vi "FPGA_HoppingScan_CircularBuffered.vi"() -> ()   [LabVIEW 2024]
uses:
  <vilib>/Platform/TimedLoop/XDataNode/timing_clust.ctl
  <vilib>/Platform/TimedLoop/XDataNode/nitl_modes.ctl
  <vilib>/Platform/TimedLoop/XDataNode/wakeup.ctl
  <vilib>/rvi/FXPMathLib/FxpDiv/subVIs/nifxpmath_Div_SimConfig.ctl
  <vilib>/rvi/Emulation/niFpgaSctlEmulationGetInTimedLoop.vi
  <vilib>/rvi/Emulation/niFpgaProcessEmulError.vi
  <vilib>/rvi/Memory/Memory_Emulation/nirvimemoryFastEmulation.vi
  <vilib>/rvi/Memory/Memory_Emulation/nirvimemoryEmulation.vi
  <vilib>/rvi/Emulation/niFpgaEmulationIsFPGAContextNoSignature.vi
  <vilib>/rvi/DataTransferAndStorage/Container/Common/niFpgaContainerGetUniqueNameForEmu.vi
  <vilib>/rvi/errors/nirviReportUnexpectedCaseInternalError (U32).vi
  <vilib>/rvi/eio/common/nirviEmuTemplateMethod_errors.vi
  <vilib>/rvi/Emulation/niFpgaEmulationReportErrorSimple.vi
  <vilib>/rvi/Emulation/niFpgaGetClockAttributes.vi
  <vilib>/rvi/Emulation/niFpgaCriticalErrorInLSC.vi
  <vilib>/rvi/Memory/Memory_Emulation/niFpgaMemoryEmulationCacheClearOnFirstRun.vi
  <vilib>/rvi/Memory/Memory_Emulation/nirvimemoryEmulationManagerCache_MakeExclusive.vi
  <vilib>/rvi/Memory/Memory_Emulation/niFpgaMemoryEmulationValidateCache.vi
  <vilib>/rvi/Memory/Memory_Emulation/nirvimemoryEmulationManagerCache_InsertValue.vi
  <vilib>/Utility/error.llb/Clear Errors.vi
  <vilib>/rvi/Memory/Memory_Emulation/nirvimemoryEmulationManagerCache_ReleaseExclusive.vi
  <vilib>/rvi/Memory/Memory_Emulation/nirvimemoryEmulationManagerCache_GetValue.vi
  <vilib>/rvi/Memory/Memory_Emulation/nirvimemoryEmulationManagerCache_SetValue.vi
  <vilib>/rvi/FIFO/Fifo_Resource/nirvififoEmulationSetSize.vi
  <vilib>/rvi/FIFO/Fifo_Resource/nirviFifoEmulationQueueMgr.vi
  <instcachedir>/0/nirviFifoEmulationQueueMgr_E5CAEC123FF24DC58D834DCA3CDAA9B5.lvgen/nirviFifoEmulationQueueMgr_E5CAEC123FF24DC58D834DCA3CDAA9B5_001.vi
  <vilib>/rvi/errors/niFpgaSetErrorForExecOnDevCompSimple.vi
  <vilib>/rvi/eio/common/nirviEmuReportErrorAndStop.vi
  <vilib>/rvi/FIFO/Fifo_Resource/nirvififoEmulationCreateLock.vi
  <vilib>/rvi/FIFO/Fifo_Resource/nirvififoEmulationObtainLock.vi
  <vilib>/rvi/FIFO/Fifo_Resource/nirvififoEmulationReleaseLock.vi
  <vilib>/rvi/occurrence/nirviWaitOnOccurrenceBase.vi
  <vilib>/rvi/errors/nirviReportUnexpectedCaseInternalError.vi
  <vilib>/eio/utilities/niEioResolveVilibRelativePath.vi
  <vilib>/rvi/interface/RandomDataEmulation/niFpgaRandomDataHandleErrors.vi
  <vilib>/rvi/FXPMathLib/FxpDiv/simVIs/DllFxpDivTemp_sub.vi
  <vilib>/rvi/FIFO/Fifo_Resource/nirvififoEmulationDetermineInputValidOut.vi
  <vilib>/rvi/DataTransferAndStorage/Container/XNode/niFpgaContainer.xnode
  <vilib>/eio/EIONode/EIONode.xnode
  <vilib>/platform/TimedLoop/XDataNode/XDataNode.xnode
  <vilib>/rvi/DataTransferAndStorage/Register/Emulation/niFpgaRegisterEmulation.vi
  <vilib>/rvi/FIFO/Fifo_Resource/nirvififoEmulationGetNumberOfElementsToRead.vi
  <vilib>/rvi/FIFO/Fifo_Resource/nirvififoEmulationRead.vi
  <vilib>/rvi/interface/RandomDataEmulation/nirviRandomDataFpgaReadWriteTemplate.vi
  <vilib>/rvi/FXPMathLib/FxpSub/XNode/nifxpmath_Sub.xnode
  <vilib>/rvi/FXPMathLib/FxpAdd/XNode/nifxpmath_Add.xnode
  <vilib>/rvi/FXPMathLib/FxpMul/XNode/nifxpmath_Multiplier.xnode
  <vilib>/rvi/FXPMathLib/FxpDiv/XNode/nifxpmath_Div.xnode
  <vilib>/rvi/FIFO/Fifo_Resource/nirvififoEmulationWrite.vi
  <vilib>/rvi/FXPMathLib/sim/FxpSim.dll
  <vilib>/Platform/TimedLoop/XDataNode/XDNodeRunTimeDep.lvlib
panel:
  in  "DelayPoints":i32
  in  "Halting Threshold":fxp<+/-,48,16>
  out "point_scanned":u32
  in  "TotalPoints":u32
  in  "RetRate us":i32
  in  "AppRate_NF us":i32
  in  "AppRate_FF us":i32
  in  "Recording Threshold":fxp<+/-,48,16>
  in  "stop":bool
  out "TargetDone?":bool
  out "ScanFinished?":bool
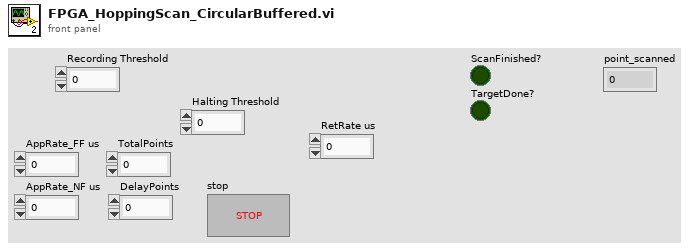
[diagram p1: front panel]
types:
  T1 = typedef "XDNodeRunTimeDep.lvlib/timing_clust.ctl" = cluster{"Expected End [f-1]":u64, "Actual End [f-1]":u64, "Finished Late? [f-1]":bool, "Expected End [i-1]":u64, "Actual End [i-1]":u64, "Finished Late? [i-1]":bool, "Expected Start [i]":u64, "Actual Start [i]":u64, "Expected Start [f]":u64, "Actual Start [f]":u64, "Source Name":string, "Structure Name":string, "Period":i64, "Deadline":i64, "Offset":i64, "Start":i64, "Priority":i32, "Timeout":i32, "Mode":T2, "Wakeup Reason":T3, "Error":errorcluster, "Source Type":string, "Secondary Source Type":string, "Global End Time":u64, "Global Start Time":u64, "Frame Duration":u64, "Iteration Duration":u64, "Assigned CPU":i32, "I/O Scan Engine Mode":u32}
  T2 = typedef "XDNodeRunTimeDep.lvlib/nitl_modes.ctl" = enum32{"No Change", "Process missed periods, maintain original phase", "Discard missed periods, maintain original phase", "Process missed periods, ignore original phase", "Discard missed periods, ignore original phase"}
  T3 = typedef "XDNodeRunTimeDep.lvlib/wakeup.ctl" = enum32{"Normal", "Aborted", "Asynchronous wakeup", "Timing source error", "Timed loop error", "Timeout"}
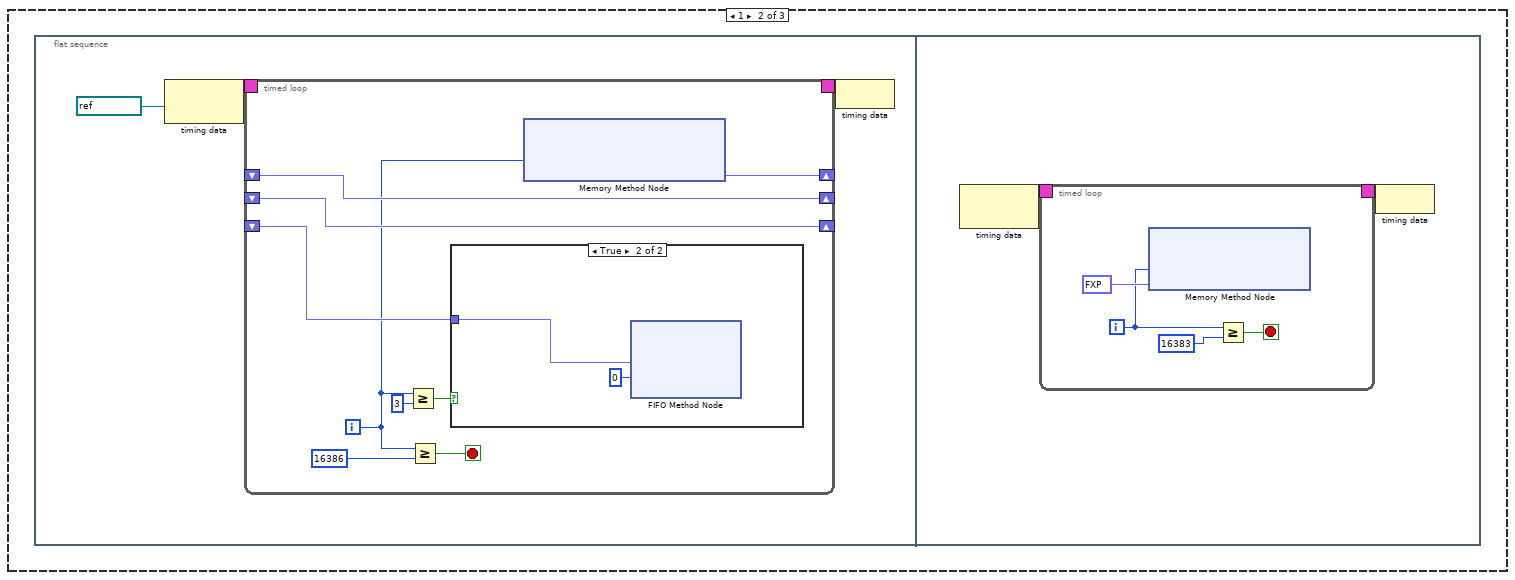
[diagram p4: hidden frame]
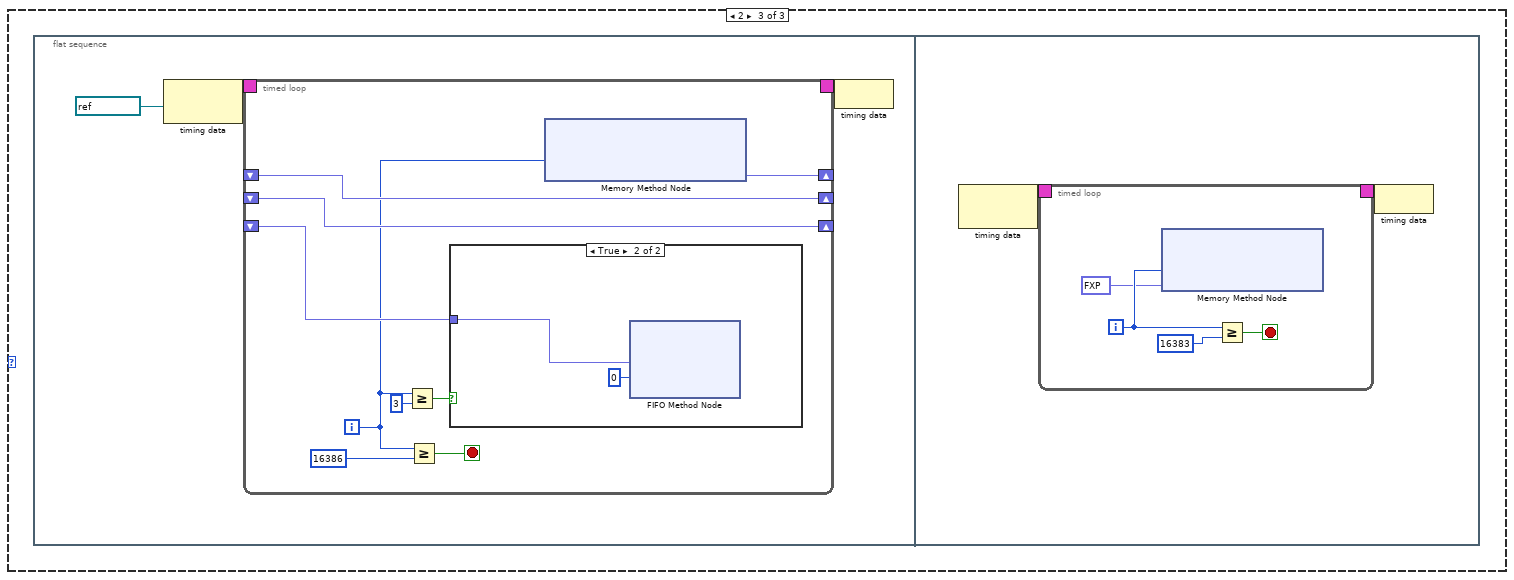
[diagram p6: hidden frame]
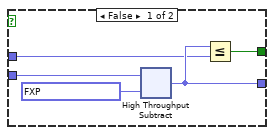
[diagram p13: hidden frame]
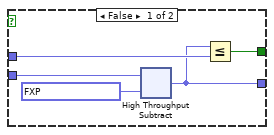
[diagram p14: hidden frame]
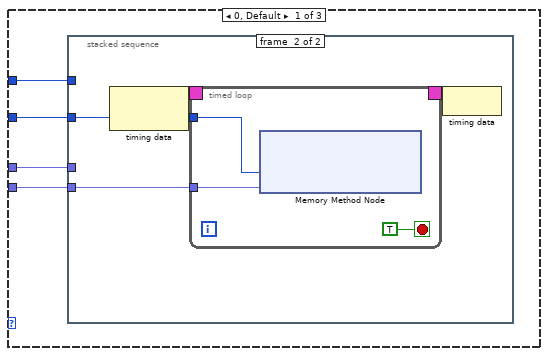
[diagram p16: hidden frame]
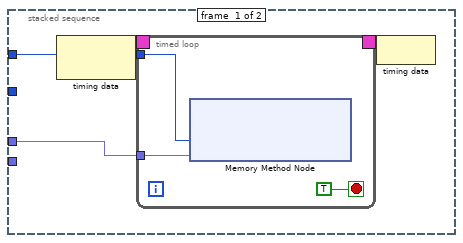
[diagram p17: hidden frame]
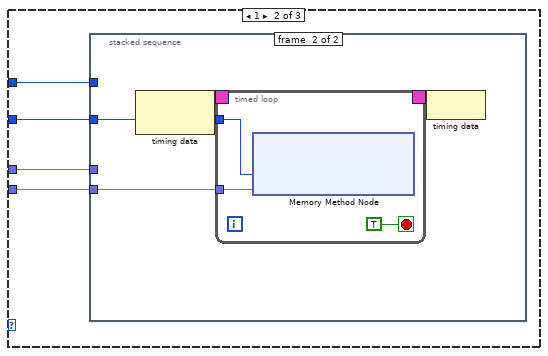
[diagram p18: hidden frame]
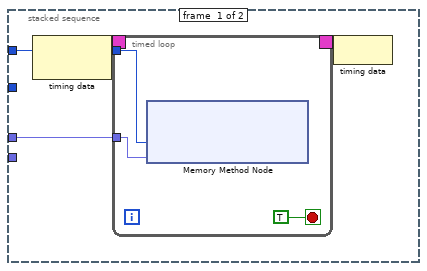
[diagram p19: hidden frame]
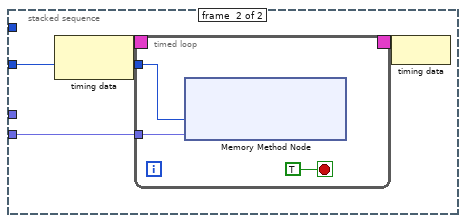
[diagram p20: hidden frame]
diagram:
  n1 = flat-sequence {
    tunnel: [w18] -> w1
    tunnel: w1 -> [w31]
    frame #0 {
      w7 = fxp<+/-,20,5> 0.0 ("Connector0/AO0")
      n2 = node-c288() -> (w3:T1)  [unwired: 1 in]
      n3 = timed-loop {
        timing: w3 -> [_]
        timing-out: [_] -> w2
        i -> [w9]
        stop <- w8 stop-if-true
        w11 = fxp<+/-,48,16> -100.0 ("Data")
        n4 = xnode ("Memory Method Node")("Address"=w9, "Data"=w11) -> ()  [unwired: 1 in, 1 out]
        n5 = xnode ("Memory Method Node")("Address"=w9, "Data"=w11) -> ()  [unwired: 1 in, 1 out]
        n6 = xnode ("Memory Method Node")("Address"=w9, "Data"=w11) -> ()  [unwired: 1 in, 1 out]
        n7 = Greater Or Equal?(x=w9, y=16383) -> (x >= y?=w8:bool)
      }
      n8 = for {
        N: 6 -> [_]
        i -> [w17]
        n9 = xnode ("Memory Method Node")("Address"=w17, "Data"=fxp<+/-,48,16> 0.0) -> ()  [unwired: 1 in, 1 out]
      }
      n10 = xnode "FPGA I/O Node"("Connector0/AO0"=w7, "Connector0/AO1"=w7, "Connector0/AO2"=w7) -> ()  [unwired: 3 in, 3 out]
      n11 = node-c288(w2) -> ()
      "ScanFinished?" <- FALSE
      "TargetDone?" <- FALSE
    }
    frame #1 {
      n12 = Generate Occurrence() -> (w18:refnum<k4>)
      n13 = call "Wait"("Count(mSec)"=u8 120) -> ()  [unwired: 1 out]
    }
    frame #2 {
      n14 = while {
        tunnel: w31 -> [w148]
        stop <- w150 stop-if-true
        n15 = xnode ("Register Read")() -> ("Data"=w151:bool)  [unwired: 1 in, 1 out]
        n16 = xnode ("FIFO Method Node")() -> ("Number of Elements to Read"=w154:u32)  [unwired: 1 in, 1 out]
        n17 = local read "ScanFinished?"() -> (w149:bool)
        n18 = Or(x=w151, y=w149) -> (x .or. y?=w150:bool)
        n19 = Greater Or Equal?(x=w154, y=u32 6) -> (x >= y?=w152:bool)
        n20 = case shown="True" w152 {
          tunnel: w148 -> [_ w155]
          frame False {
          }
          frame True {
            n21 = First Call?() -> (First Call?: T/F=w156:bool)
            n22 = case shown="True" w156 {
              tunnel: w155 -> [_ w157]
              frame False {
              }
              frame True {
                n23 = flat-sequence {
                  tunnel: [w160] -> w158
                  tunnel: w157 -> [w160]
                  tunnel: w158 -> [w161]
                  frame #0 {
                    n24 = call "Wait3"("Count(mSec)"=u8 4) -> ()  [unwired: 1 out]
                  }
                  frame #1 {
                    n25 = Set Occurrence(w161) -> ()
                  }
                }
              }
            }
          }
        }
      }
      n26 = while {
        tunnel: w31 -> [w133]
        stop <- w130 stop-if-true
        n27 = flat-sequence {
          tunnel: ["stop"] -> w135
          tunnel: w133 -> [w137]
          tunnel: [w137] -> w131
          tunnel: w135 -> [w140]
          tunnel: [w140] -> w134
          tunnel: [w139] -> w132
          tunnel: w131 -> [w139]
          tunnel: w134 -> [w144]
          tunnel: w132 -> [w143]
          tunnel: [w142] -> w130
          frame #0 {
            n28 = case shown="True" "stop" {
              tunnel: "stop" -> [_ w138]
              frame False {
              }
              frame True {
                n29 = xnode ("Register Write")("Data"=w138) -> ()  [unwired: 1 in, 1 out]
              }
            }
          }
          frame #1 {
            n30 = call "Wait2"("Count(uSec)"=u8 200) -> ()  [unwired: 1 out]
          }
          frame #2 {
            n31 = xnode ("Register Read")() -> ("Data"=w145:bool)  [unwired: 1 in, 1 out]
            n32 = local read "ScanFinished?"() -> (w146:bool)
            n33 = Compound Arithmetic op=OR(w146, w145, w144) -> (w142:bool)
            n34 = case shown="True" w142 {
              tunnel: w143 -> [_ w147]
              frame False {
              }
              frame True {
                n35 = Set Occurrence(w147) -> ()
              }
            }
          }
        }
      }
      n36 = flat-sequence {
        tunnel: w31 -> [w162]
        tunnel: [fxp<+/-,48,16> 0.0 ("Threshold")] -> w30
        tunnel: [w164] -> w28
        tunnel: [u8 0] -> w25
        tunnel: w30 -> [w167]
        tunnel: [w168] -> w29
        tunnel: w28 -> [w168]
        tunnel: [w167] -> w27
        tunnel: [w166] -> w26
        tunnel: w25 -> [w166]
        tunnel: w29 -> [w173]
        tunnel: w27 -> [w172]
        tunnel: w26 -> [w171]
        tunnel: [w170] -> w24
        tunnel: w24 -> [w1125]
        tunnel: [w1123] -> w23
        tunnel: [w1122] -> w21
        tunnel: w23 -> [w1137]
        tunnel: [w1137] -> w22
        tunnel: w21 -> [w1136]
        tunnel: [w1136] -> w20
        tunnel: w22 -> [w1141]
        tunnel: w20 -> [w1138]
        frame #0 {
          n37 = Wait on Occurrence(2:w162) -> ()  [unwired: 2 in, 1 out]
        }
        frame #1 {
          # "z piezo voltage"
          # "Swapchain indicator"
          n38 = xnode ("Register Read")() -> ("Data"=w164:bool)  [unwired: 1 in, 1 out]
        }
        frame #2 {
          n39 = call "Wait4"("Count(mSec)"=u8 4) -> ()  [unwired: 1 out]
        }
        frame #3 {
          n40 = case shown="False" w173 {
            tunnel: w172 -> [w176 w1121]
            tunnel: w171 -> [w175 _]
            tunnel: [w174 w1121] -> w170
            frame False {
              n41 = while {
                shift-right: [w184] -> w174
                shift-left: w176 -> [w218]
                shift-right: [w183] -> _
                shift-left: w175 -> [w197]
                stop <- w182 stop-if-true
                n42 = flat-sequence {
                  tunnel: w218 -> [w220]
                  tunnel: [w222] -> w217
                  tunnel: [w221] -> w213
                  tunnel: [w220] -> w202
                  tunnel: w197 -> [w219]
                  tunnel: [w219] -> w196
                  tunnel: w217 -> [w230]
                  tunnel: [w230] -> w216
                  tunnel: w213 -> [w229]
                  tunnel: [w229] -> w212
                  tunnel: w202 -> [w228]
                  tunnel: [w228] -> w201
                  tunnel: w196 -> [w227]
                  tunnel: [w227] -> w195
                  tunnel: w216 -> [w257]
                  tunnel: [w257] -> w215
                  tunnel: [w250] -> w214
                  tunnel: w212 -> [w256]
                  tunnel: [w256] -> w211
                  tunnel: [w251] -> w209
                  tunnel: [w254] -> w207
                  tunnel: [w253] -> w206
                  tunnel: [w252] -> w205
                  tunnel: w201 -> [w249]
                  tunnel: w195 -> [w255]
                  tunnel: [w255] -> w194
                  tunnel: [w246] -> w181
                  tunnel: [w248] -> w177
                  tunnel: w215 -> [w293]
                  tunnel: w214 -> [w294]
                  tunnel: w211 -> [w292]
                  tunnel: [w292] -> w210
                  tunnel: w209 -> [w291]
                  tunnel: [w291] -> w208
                  tunnel: w207 -> [w290]
                  tunnel: w206 -> [w288]
                  tunnel: w205 -> [w287]
                  tunnel: [w290] -> w204
                  tunnel: [w285] -> w200
                  tunnel: w194 -> [w289]
                  tunnel: [w289] -> w193
                  tunnel: [w288] -> w190
                  tunnel: [w287] -> w189
                  tunnel: w181 -> [w286]
                  tunnel: [w286] -> w180
                  tunnel: w177 -> [w285]
                  tunnel: w210 -> [w321]
                  tunnel: w208 -> [w322]
                  tunnel: w204 -> [w320]
                  tunnel: [w320] -> w203
                  tunnel: w200 -> [w319]
                  tunnel: [w319] -> w199
                  tunnel: w193 -> [w318]
                  tunnel: [w318] -> w191
                  tunnel: w190 -> [w317]
                  tunnel: w189 -> [w316]
                  tunnel: [w317] -> w188
                  tunnel: [w316] -> w187
                  tunnel: w180 -> [w315]
                  tunnel: [w315] -> w179
                  tunnel: w203 -> [w348]
                  tunnel: w199 -> [w347]
                  tunnel: [w347] -> w198
                  tunnel: [w346] -> w192
                  tunnel: w191 -> [w346]
                  tunnel: w188 -> [w345]
                  tunnel: w187 -> [w344]
                  tunnel: [w345] -> w186
                  tunnel: [w344] -> w185
                  tunnel: w179 -> [w343]
                  tunnel: [w343] -> w178
                  tunnel: w198 -> [w363]
                  tunnel: w192 -> [w362]
                  tunnel: w186 -> [w361]
                  tunnel: w185 -> [w360]
                  tunnel: [w359] -> w183
                  tunnel: [w358] -> w184
                  tunnel: [w357] -> w182
                  tunnel: w178 -> [w353]
                  frame #0 {
                    # "Data from target to host:\n0, 1: X, Y piezo voltage\n2, 3: X, Y piezo idx\n4: Z piezo voltage\n5: baseline current\n6: circular buffer pointer idx\n(7-8106): Z voltage\n(8107-16206): current"
                    # "Data from host to target:\n0, 1: X, Y piezo voltage\n2, 3: X, Y piezo idx\n4: distance (piezo voltage) to the last point\n5: retract height, \nall negative cases won't trigger approach of z piezo\nif -20, keep z and move xy\nif -30, full retract for z and move xy"
                    n43 = for {
                      N: 2 -> [_]
                      shift-right: [w226] -> w221
                      shift-left: _ -> [w224]
                      shift-right: [w224] -> w222
                      shift-left: _ -> [_]
                      i -> [w225]
                      n44 = xnode ("Memory Method Node")("Address"=w225) -> ("Data"=w226:fxp<+/-,48,16>)  [unwired: 1 in, 1 out]
                    }
                  }
                  frame #1 {
                    # "y"
                    # "x"
                    n45 = while {
                      shift-right: [w234] -> _
                      shift-left: i16 0 -> [w233]
                      stop <- w235 stop-if-true
                      n46 = xnode ("FIFO Method Node")("Timeout"=8192) -> ("Element"=w232:fxp<+/-,48,16>, "Timed Out?"=w239:bool)  [unwired: 1 in, 1 out]
                      n47 = Increment(x=w233) -> (x+1=w242:i16)
                      n48 = xnode ("Register Read")() -> ("Data"=w236:bool)  [unwired: 1 in, 1 out]
                      n49 = Select(t=w233, s=w239, f=w242) -> (s? t:f=w234:i16)
                      n50 = Not(x=w239) -> (.not. x?=w238:bool)
                      n51 = Equal?(x=w233, y=i16 5) -> (x = y?=w240:bool)
                      n52 = And(x=w240, y=w238) -> (x .and. y?=w237:bool)
                      n53 = xnode ("Memory Method Node")("Address"=w233, "Data"=w232) -> ()  [unwired: 1 in, 1 out]
                      n54 = Or(x=w237, y=w236) -> (x .or. y?=w235:bool)
                    }
                  }
                  frame #2 {
                    # "0"
                    # "5"
                    n55 = for {
                      N: 6 -> [_]
                      shift-right: [w283] -> w246
                      shift-left: _ -> [w282]
                      shift-right: [w282] -> w254
                      shift-left: _ -> [w281]
                      shift-right: [w281] -> w253
                      shift-left: _ -> [w280]
                      shift-right: [w280] -> w252
                      shift-left: _ -> [w279]
                      shift-right: [w279] -> w251
                      shift-left: _ -> [w278]
                      shift-right: [w278] -> w250
                      shift-left: _ -> [_]
                      i -> [w284]
                      n56 = xnode ("Memory Method Node")("Address"=w284) -> ("Data"=w283:fxp<+/-,48,16>)  [unwired: 1 in, 1 out]
                    }
                    n57 = Equal?(x=w246, y=fxp<+/-,48,16> -30.0) -> (x = y?=w245:bool)
                    n58 = case shown="True" w245 {
                      tunnel: w249 -> [w259 w263]
                      tunnel: [w259 w262] -> w248
                      tunnel: fxp<+/-,48,16> 0.0048828125 ("y") -> [_ w261]
                      frame False {
                      }
                      frame True {
                        n59 = flat-sequence {
                          tunnel: w263 -> [w266]
                          tunnel: w261 -> [w264]
                          tunnel: [w265] -> w260
                          tunnel: [w277] -> w262
                          tunnel: w260 -> [w277]
                          frame #0 {
                            n60 = while {
                              shift-right: [w270] -> w265
                              shift-left: w266 -> [w275]
                              tunnel: w264 -> [w269]
                              stop <- w271 stop-if-true
                              w272 = fxp<+/-,48,16> 0.0 ("y")
                              n61 = xnode "High Throughput Subtract"("x"=w275, "y"=w269) -> ("x-y"=w273:fxp<+/-,48,16>)
                              n62 = xnode ("Register Read")() -> ("Data"=w274:bool)  [unwired: 1 in, 1 out]
                              n63 = Less Or Equal?(x=w273, y=w272) -> (x <= y?=w267:bool)
                              n64 = Select(t=w272, s=w267, f=w273) -> (s? t:f=w270:fxp<+/-,48,16>)
                              n65 = local read "RetRate us"() -> (w268:i32)
                              n66 = xnode "FPGA I/O Node"("Connector0/AO2"=w270) -> ()  [unwired: 1 in, 1 out]
                              n67 = Compound Arithmetic op=OR(w267, w274) -> (w271:bool)
                              n68 = call "Wait10"("Count(uSec)"=w268) -> ()  [unwired: 1 out]
                            }
                          }
                          frame #1 {
                            n69 = call "Wait17"("Count(mSec)"=u16 2 ("Count(uSec)")) -> ()  [unwired: 1 out]
                          }
                        }
                      }
                    }
                  }
                  frame #3 {
                    n70 = xnode "High Throughput Subtract"("x"=w293, "y"=w294) -> ("x-y"=w296:fxp<+/-,48,16>)
                    n71 = Less Or Equal To 0?(x=w296) -> (x <= 0?=w295:bool)
                    n72 = while {
                      tunnel: w295 -> [w304]
                      tunnel: w294 -> [w303]
                      shift-right: [w297] -> _
                      shift-left: w293 -> [w299]
                      stop <- w300 stop-if-true
                      n73 = case shown="True" w304 {
                        tunnel: w303 -> [w305 w310]
                        tunnel: w299 -> [w308 w314]
                        tunnel: [w307 w312] -> w298
                        tunnel: [w306 w311] -> w297
                        frame False {
                          n74 = xnode "High Throughput Subtract"("x"=w308, "y"=fxp<+/-,48,16> 0.00030517578125) -> ("x-y"=w306:fxp<+/-,48,16>)
                          n75 = Less Or Equal?(x=w306, y=w305) -> (x <= y?=w307:bool)
                        }
                        frame True {
                          n76 = xnode ("High Throughput Add")("x"=w314, "y"=fxp<+/-,48,16> 0.00030517578125) -> ("x+y"=w311:fxp<+/-,48,16>)
                          n77 = Greater Or Equal?(x=w311, y=w310) -> (x >= y?=w312:bool)
                        }
                      }
                      n78 = call "Wait5"("Count(uSec)"=u32 70) -> ()  [unwired: 1 out]
                      n79 = xnode ("Register Read")() -> ("Data"=w301:bool)  [unwired: 1 in, 1 out]
                      n80 = xnode "FPGA I/O Node"("Connector0/AO0"=w297) -> ()  [unwired: 1 in, 1 out]
                      n81 = Or(x=w298, y=w301) -> (x .or. y?=w300:bool)
                    }
                  }
                  frame #4 {
                    n82 = xnode "High Throughput Subtract"("x"=w321, "y"=w322) -> ("x-y"=w324:fxp<+/-,48,16>)
                    n83 = Less Or Equal To 0?(x=w324) -> (x <= 0?=w323:bool)
                    n84 = while {
                      tunnel: w323 -> [w332]
                      tunnel: w322 -> [w331]
                      shift-right: [w325] -> _
                      shift-left: w321 -> [w327]
                      stop <- w328 stop-if-true
                      n85 = case shown="True" w332 {
                        tunnel: w331 -> [w334 w339]
                        tunnel: w327 -> [w336 w342]
                        tunnel: [w335 w340] -> w326
                        tunnel: [w333 w338] -> w325
                        frame False {
                          n86 = xnode "High Throughput Subtract"("x"=w336, "y"=fxp<+/-,48,16> 0.00030517578125) -> ("x-y"=w333:fxp<+/-,48,16>)
                          n87 = Less Or Equal?(x=w333, y=w334) -> (x <= y?=w335:bool)
                        }
                        frame True {
                          n88 = xnode ("High Throughput Add")("x"=w342, "y"=fxp<+/-,48,16> 0.00030517578125) -> ("x+y"=w338:fxp<+/-,48,16>)
                          n89 = Greater Or Equal?(x=w338, y=w339) -> (x >= y?=w340:bool)
                        }
                      }
                      n90 = call "Wait6"("Count(uSec)"=u32 70) -> ()  [unwired: 1 out]
                      n91 = xnode ("Register Read")() -> ("Data"=w329:bool)  [unwired: 1 in, 1 out]
                      n92 = xnode "FPGA I/O Node"("Connector0/AO1"=w325) -> ()  [unwired: 1 in, 1 out]
                      n93 = Or(x=w326, y=w329) -> (x .or. y?=w328:bool)
                    }
                  }
                  frame #5 {
                    n94 = xnode ("High Throughput Multiply")("x"=w348, "y"=fxp<+/-,48,16> 1600.0) -> ("x*y"=w350:fxp<+/-,52,20>)
                    n95 = To Unsigned Long Integer(number=w350) -> (unsigned 32bit integer=w351:u32)
                    n96 = call "Wait7"("Count(uSec)"=w351) -> ()  [unwired: 1 out]
                  }
                  frame #6 {
                    # "Y, X idx"
                    n97 = xnode ("Register Read")() -> ("Data"=w356:bool)  [unwired: 1 in, 1 out]
                    n98 = Less Or Equal?(x=w353, y=fxp<+/-,48,16> -20.0) -> (x <= y?=w354:bool)
                    n99 = Or(x=w354, y=w356) -> (x .or. y?=w355:bool)
                    n100 = case shown="False" w355 {
                      tunnel: w363 -> [w383 w1120]
                      tunnel: w362 -> [w381 w1119]
                      tunnel: w361 -> [w375 _]
                      tunnel: w360 -> [w374 _]
                      tunnel: [w372 w1120] -> w358
                      tunnel: [w373 w1119] -> w359
                      tunnel: [w371 w1116] -> w357
                      tunnel: w354 -> [_ w1118]
                      tunnel: w353 -> [w367 _]
                      frame False {
                        n101 = flat-sequence {
                          tunnel: [w389] -> w386
                          tunnel: [w394] -> w385
                          tunnel: [w393] -> w384
                          tunnel: w383 -> [w392]
                          tunnel: [w392] -> w382
                          tunnel: w381 -> [w391]
                          tunnel: [w391] -> w380
                          tunnel: [0] -> w379
                          tunnel: [w389] -> w366
                          tunnel: [FALSE] -> w364
                          tunnel: w386 -> [w440]
                          tunnel: w385 -> [w439]
                          tunnel: w384 -> [w438]
                          tunnel: w382 -> [w437]
                          tunnel: w380 -> [w436]
                          tunnel: w379 -> [w431]
                          tunnel: [w435] -> w378
                          tunnel: [w434] -> w377
                          tunnel: [w433] -> w376
                          tunnel: w366 -> [w432]
                          tunnel: [w432] -> w365
                          tunnel: w364 -> [w430]
                          tunnel: w378 -> [w770]
                          tunnel: w377 -> [w772]
                          tunnel: w376 -> [w773]
                          tunnel: w375 -> [w775]
                          tunnel: w374 -> [w774]
                          tunnel: [w771] -> w370
                          tunnel: [w770] -> w369
                          tunnel: [w767] -> w368
                          tunnel: w365 -> [w766]
                          tunnel: [w1096] -> w371
                          tunnel: [w1095] -> w372
                          tunnel: [w1097] -> w373
                          tunnel: w370 -> [w1097]
                          tunnel: w369 -> [w1092]
                          tunnel: w368 -> [w1096]
                          tunnel: w367 -> [w1093]
                          frame #0 {
                            n102 = for {
                              N: 32 -> [_]
                              shift-right: [w427] -> w397
                              shift-left: fxp<+/-,48,16> 0.0 -> [w428]
                              n103 = xnode "FPGA I/O Node"() -> ("Connector0/AI3"=w429:fxp<+/-,27,5>)  [unwired: 1 in, 1 out]
                              n104 = xnode ("High Throughput Add")("x"=w429, "y"=w428) -> ("x+y"=w427:fxp<+/-,48,16>)
                            }
                            n105 = local read "Halting Threshold"() -> (w388:fxp<+/-,48,16>)
                            n106 = local read "Recording Threshold"() -> (w395:fxp<+/-,48,16>)
                            n107 = xnode "High Throughput Divide"("x"=w397, "y"=fxp<+/-,48,16> 32.0) -> ("x/y"=w389:fxp<+/-,48,16>)
                            n108 = xnode ("High Throughput Multiply")("x"=w389, "y"=w395) -> ("x*y"=w394:fxp<+/-,48,16>)
                            n109 = xnode ("High Throughput Multiply")("x"=w389, "y"=w388) -> ("x*y"=w393:fxp<+/-,48,16>)
                          }
                          frame #1 {
                            n110 = while {
                              tunnel: w440 -> [w503]
                              tunnel: w439 -> [w502]
                              tunnel: w438 -> [w501]
                              shift-right: [w480] -> w435
                              shift-left: w437 -> [w500]
                              shift-right: [w479] -> w434
                              shift-left: w436 -> [w499]
                              shift-right: [w462] -> _
                              shift-left: w431 -> [w498]
                              shift-right: [w463] -> _
                              shift-left: w431 -> [w487]
                              tunnel: [w473] -> w433
                              shift-right: [w447] -> _
                              shift-left: w431 -> [w451]
                              shift-right: [w441] -> _
                              shift-left: w430 -> [w445]
                              stop <- w476 stop-if-true
                              n111 = flat-sequence {
                                tunnel: w487 -> [w507]
                                tunnel: w498 -> [w508]
                                tunnel: w499 -> [w509]
                                tunnel: w500 -> [w510]
                                tunnel: w501 -> [w511]
                                tunnel: w502 -> [w512]
                                tunnel: w503 -> [w513]
                                tunnel: [w513] -> w472
                                tunnel: [w512] -> w471
                                tunnel: [w511] -> w470
                                tunnel: [w510] -> w469
                                tunnel: [w509] -> w468
                                tunnel: [w508] -> w467
                                tunnel: [w507] -> w466
                                tunnel: [w506] -> w465
                                tunnel: [w505] -> w452
                                tunnel: w451 -> [w505]
                                tunnel: [w504] -> w446
                                tunnel: w445 -> [w504]
                                tunnel: [w561] -> w497
                                tunnel: [w557] -> w496
                                tunnel: [w556] -> w495
                                tunnel: [w544] -> w491
                                tunnel: [w541] -> w490
                                tunnel: [w555] -> w486
                                tunnel: [w554] -> w484
                                tunnel: [w553] -> w481
                                tunnel: [w534] -> w478
                                tunnel: [w546] -> w474
                                tunnel: w472 -> [w568]
                                tunnel: w471 -> [w566]
                                tunnel: w470 -> [w536]
                                tunnel: w469 -> [w558]
                                tunnel: w468 -> [w554]
                                tunnel: w467 -> [w531]
                                tunnel: w466 -> [w555]
                                tunnel: w465 -> [w540]
                                tunnel: [w540] -> w464
                                tunnel: w452 -> [w520]
                                tunnel: [w521] -> w449
                                tunnel: w446 -> [w517]
                                tunnel: [w515] -> w444
                                tunnel: w497 -> [w640]
                                tunnel: w496 -> [w639]
                                tunnel: w495 -> [w641]
                                tunnel: [w641] -> w494
                                tunnel: [w640] -> w493
                                tunnel: [w639] -> w492
                                tunnel: w491 -> [w638]
                                tunnel: w490 -> [w637]
                                tunnel: [w638] -> w489
                                tunnel: [w637] -> w488
                                tunnel: w486 -> [w636]
                                tunnel: [w636] -> w485
                                tunnel: w484 -> [w635]
                                tunnel: [w635] -> w483
                                tunnel: [w634] -> w482
                                tunnel: w481 -> [w634]
                                tunnel: w478 -> [w633]
                                tunnel: [w633] -> w477
                                tunnel: [w632] -> w475
                                tunnel: w474 -> [w632]
                                tunnel: w464 -> [w631]
                                tunnel: [w631] -> w455
                                tunnel: [w630] -> w450
                                tunnel: w449 -> [w630]
                                tunnel: w444 -> [w629]
                                tunnel: [w629] -> w443
                                tunnel: w494 -> [w652]
                                tunnel: w493 -> [w663]
                                tunnel: w492 -> [w656]
                                tunnel: w489 -> [w658]
                                tunnel: w488 -> [w657]
                                tunnel: w485 -> [w644]
                                tunnel: w483 -> [w655]
                                tunnel: w482 -> [w646]
                                tunnel: w477 -> [w654]
                                tunnel: w475 -> [w653]
                                tunnel: [w663] -> w461
                                tunnel: [w659] -> w460
                                tunnel: [w656] -> w459
                                tunnel: [w655] -> w458
                                tunnel: [w654] -> w457
                                tunnel: [w653] -> w456
                                tunnel: w455 -> [w650]
                                tunnel: [w650] -> w454
                                tunnel: [w649] -> w453
                                tunnel: w450 -> [w648]
                                tunnel: [w648] -> w448
                                tunnel: w443 -> [w647]
                                tunnel: [w647] -> w442
                                tunnel: [w760] -> w473
                                tunnel: [w761] -> w476
                                tunnel: [w762] -> w479
                                tunnel: [w763] -> w480
                                tunnel: [w764] -> w463
                                tunnel: [w765] -> w462
                                tunnel: w461 -> [w765]
                                tunnel: w460 -> [w764]
                                tunnel: w459 -> [w763]
                                tunnel: w458 -> [w762]
                                tunnel: w457 -> [w761]
                                tunnel: w456 -> [w760]
                                tunnel: w454 -> [w758]
                                tunnel: w453 -> [w757]
                                tunnel: [w751] -> w447
                                tunnel: w448 -> [w751]
                                tunnel: w442 -> [w750]
                                tunnel: [w750] -> w441
                                frame #0 {
                                n112 = call "Tick Count"() -> ("Tick Count(uSec)"=w506:u32)
                                }
                                frame #1 {
                                w518 = 16
                                w533 = 1 ("y")
                                w559 = fxp<+/-,48,16> 0.0 ("y")
                                # "brake zone"
                                # "recording zone"
                                # "speed switch"
                                n113 = for {
                                N: w518 -> [_]
                                shift-right: [w626] -> w545
                                shift-left: w559 -> [w627]
                                shift-right: [w623] -> w543
                                shift-left: w559 -> [w625]
                                n114 = xnode "FPGA I/O Node"() -> ("Connector0/AI2"=w628:fxp<+/-,27,5>, "Connector0/AI3"=w624:fxp<+/-,27,5>)  [unwired: 2 in, 2 out]
                                n115 = xnode ("High Throughput Add")("x"=w625, "y"=w624) -> ("x+y"=w623:fxp<+/-,48,16>)
                                n116 = xnode ("High Throughput Add")("x"=w628, "y"=w627) -> ("x+y"=w626:fxp<+/-,48,16>)
                                }
                                n117 = To Fixed-Point(number=w518) -> (fixed-point=w542:fxp<+/-,48,16>)  [unwired: 1 in]
                                n118 = local read "DelayPoints"() -> (w514:i32)
                                n119 = Not Equal To 0?(x=w520) -> (x != 0?=w519:bool)
                                n120 = Greater Or Equal?(x=w520, y=w514) -> (x >= y?=w527:bool)
                                n121 = Select(t=fxp<+/-,48,16> 0.0 ("y"), s=w519, f=fxp<+/-,48,16> 0.00030517578125 ("y")) -> (s? t:f=w528:fxp<+/-,48,16>)
                                n122 = xnode "High Throughput Divide"("x"=w545, "y"=w542) -> ("x/y"=w544:fxp<+/-,48,16>)
                                n123 = xnode "High Throughput Divide"("x"=w543, "y"=w542) -> ("x/y"=w541:fxp<+/-,48,16>)
                                n124 = xnode ("High Throughput Add")("x"=w528, "y"=w558) -> ("x+y"=w547:fxp<+/-,48,16>)
                                n125 = xnode "High Throughput Subtract"("x"=w568, "y"=w541) -> ("x-y"=w567:fxp<+/-,48,16>)
                                n126 = Absolute Value(x=w567) -> (abs(x)=w537:fxp<+,48,16>)
                                n127 = Less Or Equal?(x=w547, y=fxp<+/-,48,16> 9.75) -> (x <= y?=w549:bool)
                                n128 = Greater Or Equal?(x=w547, y=fxp<+/-,48,16> -0.125) -> (x >= y?=w550:bool)
                                n129 = And(x=w550, y=w549) -> (x .and. y?=w548:bool)
                                n130 = Greater Or Equal?(x=w537, y=w566) -> (x >= y?=w565:bool)
                                n131 = Less Or Equal?(x=w537, y=w536) -> (x <= y?=w539:bool)
                                n132 = Increment(x=w531) -> (x+1=w564:i32)
                                n133 = Select(t=w564, s=w565, f=0) -> (s? t:f=w561:i32)
                                n134 = xnode ("Register Read")() -> ("Data"=w553:bool)  [unwired: 1 in, 1 out]
                                n135 = Greater Or Equal?(x=w561, y=w533) -> (x >= y?=w516:bool)
                                n136 = Equal?(x=w561, y=0 ("f")) -> (x = y?=w560:bool)
                                n137 = Not(x=w539) -> (.not. x?=w546:bool)
                                n138 = Or(x=w517, y=w516) -> (x .or. y?=w515:bool)
                                n139 = Select(t=1 ("y"), s=w515, f=0) -> (s? t:f=w523:i32)
                                n140 = Add(x=w520, y=w523) -> (x+y=w522:i32)
                                n141 = Select(t=0, s=w527, f=w522) -> (s? t:f=w521:i32)
                                n142 = Greater Or Equal?(x=w561, y=w533) -> (x >= y?=w556:bool)
                                n143 = Compound Arithmetic op=AND(w539, invert w553, w548) -> (w535:bool)
                                n144 = Or(x=w560, y=w515) -> (x .or. y?=w532:bool)
                                n145 = And(x=w532, y=w535) -> (x .and. y?=w538:bool)
                                n146 = Not(x=w535) -> (.not. x?=w534:bool)
                                n147 = Select(t=w547, s=w538, f=w558) -> (s? t:f=w557:fxp<+/-,48,16>)
                                }
                                frame #2 {
                                n148 = xnode "FPGA I/O Node"("Connector0/AO2"=w639) -> ()  [unwired: 1 in, 1 out]
                                }
                                frame #3 {
                                n149 = Not(x=w646) -> (.not. x?=w645:bool)
                                n150 = Less?(x=w644, y=8099 ("f")) -> (x < y?=w642:bool)
                                n151 = case shown="True" w645 {
                                tunnel: w655 -> [_ w671]
                                tunnel: w644 -> [_ w667]
                                tunnel: w658 -> [_ w665]
                                tunnel: w657 -> [_ w664]
                                frame False {
                                }
                                frame True {
                                n152 = Add(x=w667, y=7) -> (x+y=w669:i32)
                                n153 = Add(x=w667, y=8107) -> (x+y=w666:i32)
                                n154 = case shown="2" w671 {
                                tunnel: w669 -> [w675 w699 w727]
                                tunnel: w666 -> [w674 w698 w726]
                                tunnel: w665 -> [w673 w700 w725]
                                tunnel: w664 -> [w672 w701 w724]
                                frame 0, Default {
                                n155 = stacked-sequence {
                                tunnel: w675 -> [w679 _]
                                tunnel: w674 -> [_ w690]
                                tunnel: w673 -> [w678 _]
                                tunnel: w672 -> [_ w689]
                                frame #0 {
                                n156 = node-c288() -> (w677:T1)  [unwired: 1 in]
                                n157 = timed-loop {
                                timing: w677 -> [_]
                                timing-out: [_] -> w676
                                tunnel: w679 -> [w682]
                                tunnel: w678 -> [w681]
                                stop <- TRUE stop-if-true
                                n158 = xnode ("Memory Method Node")("Address"=w682, "Data"=w681) -> ()  [unwired: 1 in, 1 out]
                                }
                                n159 = node-c288(w676) -> ()
                                }
                                frame #1 {
                                n160 = node-c288() -> (w688:T1)  [unwired: 1 in]
                                n161 = timed-loop {
                                timing: w688 -> [_]
                                timing-out: [_] -> w687
                                tunnel: w690 -> [w693]
                                tunnel: w689 -> [w692]
                                stop <- TRUE stop-if-true
                                n162 = xnode ("Memory Method Node")("Address"=w693, "Data"=w692) -> ()  [unwired: 1 in, 1 out]
                                }
                                n163 = node-c288(w687) -> ()
                                }
                                }
                                }
                                frame 1 {
                                n164 = stacked-sequence {
                                tunnel: w701 -> [_ w716]
                                tunnel: w700 -> [w705 _]
                                tunnel: w699 -> [w704 _]
                                tunnel: w698 -> [_ w715]
                                frame #0 {
                                n165 = node-c288() -> (w703:T1)  [unwired: 1 in]
                                n166 = timed-loop {
                                timing: w703 -> [_]
                                timing-out: [_] -> w702
                                tunnel: w705 -> [w708]
                                tunnel: w704 -> [w707]
                                stop <- TRUE stop-if-true
                                n167 = xnode ("Memory Method Node")("Address"=w707, "Data"=w708) -> ()  [unwired: 1 in, 1 out]
                                }
                                n168 = node-c288(w702) -> ()
                                }
                                frame #1 {
                                n169 = node-c288() -> (w714:T1)  [unwired: 1 in]
                                n170 = timed-loop {
                                timing: w714 -> [_]
                                timing-out: [_] -> w713
                                tunnel: w716 -> [w719]
                                tunnel: w715 -> [w718]
                                stop <- TRUE stop-if-true
                                n171 = xnode ("Memory Method Node")("Address"=w718, "Data"=w719) -> ()  [unwired: 1 in, 1 out]
                                }
                                n172 = node-c288(w713) -> ()
                                }
                                }
                                }
                                frame 2 {
                                n173 = stacked-sequence {
                                tunnel: w724 -> [_ w742]
                                tunnel: w725 -> [w731 _]
                                tunnel: w727 -> [w730 _]
                                tunnel: w726 -> [_ w741]
                                frame #0 {
                                n174 = node-c288() -> (w729:T1)  [unwired: 1 in]
                                n175 = timed-loop {
                                timing: w729 -> [_]
                                timing-out: [_] -> w728
                                tunnel: w731 -> [w732]
                                tunnel: w730 -> [w733]
                                stop <- TRUE stop-if-true
                                n176 = xnode ("Memory Method Node")("Address"=w733, "Data"=w732) -> ()  [unwired: 1 in, 1 out]
                                }
                                n177 = node-c288(w728) -> ()
                                }
                                frame #1 {
                                n178 = node-c288() -> (w740:T1)  [unwired: 1 in]
                                n179 = timed-loop {
                                timing: w740 -> [_]
                                timing-out: [_] -> w739
                                tunnel: w742 -> [w743]
                                tunnel: w741 -> [w744]
                                stop <- TRUE stop-if-true
                                n180 = xnode ("Memory Method Node")("Address"=w744, "Data"=w743) -> ()  [unwired: 1 in, 1 out]
                                }
                                n181 = node-c288(w739) -> ()
                                }
                                }
                                }
                                }
                                }
                                }
                                n182 = local read "AppRate_NF us"() -> (w662:i32)
                                n183 = local read "AppRate_FF us"() -> (w661:i32)
                                n184 = Increment(x=w644) -> (x+1=w660:i32)
                                n185 = Select(t=w662, s=w652, f=w661) -> (s? t:f=w649:i32)
                                n186 = Select(t=w660, s=w642, f=0) -> (s? t:f=w659:i32)
                                }
                                frame #4 {
                                n187 = call "Tick Count2"() -> ("Tick Count(uSec)"=w759:u32)
                                n188 = Subtract(x=w759, y=w758) -> (x-y=w756:i32)
                                n189 = Subtract(x=w757, y=w756) -> (x-y=w755:i32)
                                n190 = In Range and Coerce(upper limit=80000, x=w755, lower limit=1) -> (coerced(x)=w752:i32)  [unwired: 1 out]
                                n191 = call "Wait9"("Count(uSec)"=w752) -> ()  [unwired: 1 out]
                                }
                              }
                            }
                          }
                          frame #2 {
                            n192 = xnode ("Register Read")() -> ("Data"=w769:bool)  [unwired: 1 in, 1 out]
                            n193 = Compound Arithmetic op=AND(w773, invert w769) -> (w776:bool)
                            n194 = case shown="True" w776 {
                              tunnel: w775 -> [_ w796]
                              tunnel: w774 -> [_ w797]
                              tunnel: w772 -> [w778 w795]
                              tunnel: [w778 w794] -> w771
                              tunnel: [FALSE w790] -> w768
                              tunnel: w766 -> [_ w789]
                              frame False {
                              }
                              frame True {
                                w798 = fxp<+/-,48,16> 0.0 ("ZPeizoOffset")
                                n195 = for {
                                N: 16 -> [_]
                                shift-right: [w1084] -> w787
                                shift-left: w798 -> [w1088]
                                shift-right: [w1083] -> w784
                                shift-left: w798 -> [w1086]
                                shift-right: [w1080] -> w781
                                shift-left: w798 -> [w1082]
                                n196 = xnode "FPGA I/O Node"() -> ("Connector0/AI0"=w1087:fxp<+/-,27,5>, "Connector0/AI1"=w1085:fxp<+/-,27,5>, "Connector0/AI2"=w1081:fxp<+/-,27,5>)  [unwired: 3 in, 3 out]
                                n197 = xnode ("High Throughput Add")("x"=w1087, "y"=w1088) -> ("x+y"=w1084:fxp<+/-,48,16>)
                                n198 = xnode ("High Throughput Add")("x"=w1082, "y"=w1081) -> ("x+y"=w1080:fxp<+/-,48,16>)
                                n199 = xnode ("High Throughput Add")("x"=w1085, "y"=w1086) -> ("x+y"=w1083:fxp<+/-,48,16>)
                                }
                                n200 = feedback #1(u32 0 ("Timeout")) -> (w792:u32)
                                n201 = Increment(x=w792) -> (x+1=w779:u32)
                                "point_scanned" <- w779
                                n202 = feedback-in #1(w779) -> ()
                                n203 = local read "TotalPoints"() -> (w791:u32)
                                n204 = Greater Or Equal?(x=w779, y=w791) -> (x >= y?=w790:bool)
                                n205 = xnode "High Throughput Divide"("x"=w784, "y"=fxp<+/-,48,16> 16.0 ("ZPeizoOffset")) -> ("x/y"=w783:fxp<+/-,48,16>)
                                n206 = xnode "High Throughput Divide"("x"=w787, "y"=fxp<+/-,48,16> 16.0 ("ZPeizoOffset")) -> ("x/y"=w786:fxp<+/-,48,16>)
                                n207 = xnode "High Throughput Divide"("x"=w781, "y"=fxp<+/-,48,16> 16.0 ("ZPeizoOffset")) -> ("x/y"=w780:fxp<+/-,48,16>)
                                n208 = stacked-sequence {
                                tunnel: w786 -> [w881 _ _ _ _ _ _]
                                tunnel: w783 -> [_ w913 _ _ _ _ _]
                                tunnel: w780 -> [_ _ _ _ w1009 _ _]
                                tunnel: w797 -> [_ _ w946 _ _ _ _]
                                tunnel: w796 -> [_ _ _ w978 _ _ _]
                                tunnel: w795 -> [w882 w914 w945 w977 w1010 w1042 w1077]
                                tunnel: [_ _ _ _ _ _ w1075] -> w794
                                tunnel: w789 -> [_ _ _ _ _ w1041 _]
                                frame #0 {
                                n209 = case shown="2" w882 {
                                tunnel: w881 -> [w885 w895 w903]
                                frame 0, Default {
                                n210 = node-c288() -> (w884:T1)  [unwired: 1 in]
                                n211 = timed-loop {
                                timing: w884 -> [_]
                                timing-out: [_] -> w883
                                tunnel: w885 -> [w887]
                                stop <- TRUE stop-if-true
                                n212 = xnode ("Memory Method Node")("Address"=u32 0, "Data"=w887) -> ()  [unwired: 1 in, 1 out]
                                }
                                n213 = node-c288(w883) -> ()
                                }
                                frame 1 {
                                n214 = node-c288() -> (w894:T1)  [unwired: 1 in]
                                n215 = timed-loop {
                                timing: w894 -> [_]
                                timing-out: [_] -> w893
                                tunnel: w895 -> [w897]
                                stop <- TRUE stop-if-true
                                n216 = xnode ("Memory Method Node")("Address"=u32 0, "Data"=w897) -> ()  [unwired: 1 in, 1 out]
                                }
                                n217 = node-c288(w893) -> ()
                                }
                                frame 2 {
                                n218 = node-c288() -> (w905:T1)  [unwired: 1 in]
                                n219 = timed-loop {
                                timing: w905 -> [_]
                                timing-out: [_] -> w904
                                tunnel: w903 -> [w906]
                                stop <- TRUE stop-if-true
                                n220 = xnode ("Memory Method Node")("Address"=u32 0, "Data"=w906) -> ()  [unwired: 1 in, 1 out]
                                }
                                n221 = node-c288(w904) -> ()
                                }
                                }
                                }
                                frame #1 {
                                n222 = case shown="2" w914 {
                                tunnel: w913 -> [w917 w927 w935]
                                frame 0, Default {
                                n223 = node-c288() -> (w916:T1)  [unwired: 1 in]
                                n224 = timed-loop {
                                timing: w916 -> [_]
                                timing-out: [_] -> w915
                                tunnel: w917 -> [w919]
                                stop <- TRUE stop-if-true
                                n225 = xnode ("Memory Method Node")("Address"=u32 1, "Data"=w919) -> ()  [unwired: 1 in, 1 out]
                                }
                                n226 = node-c288(w915) -> ()
                                }
                                frame 1 {
                                n227 = node-c288() -> (w926:T1)  [unwired: 1 in]
                                n228 = timed-loop {
                                timing: w926 -> [_]
                                timing-out: [_] -> w925
                                tunnel: w927 -> [w929]
                                stop <- TRUE stop-if-true
                                n229 = xnode ("Memory Method Node")("Address"=u32 1, "Data"=w929) -> ()  [unwired: 1 in, 1 out]
                                }
                                n230 = node-c288(w925) -> ()
                                }
                                frame 2 {
                                n231 = node-c288() -> (w937:T1)  [unwired: 1 in]
                                n232 = timed-loop {
                                timing: w937 -> [_]
                                timing-out: [_] -> w936
                                tunnel: w935 -> [w938]
                                stop <- TRUE stop-if-true
                                n233 = xnode ("Memory Method Node")("Address"=u32 0, "Data"=w938) -> ()  [unwired: 1 in, 1 out]
                                }
                                n234 = node-c288(w936) -> ()
                                }
                                }
                                }
                                frame #2 {
                                n235 = case shown="2" w945 {
                                tunnel: w946 -> [w949 w959 w967]
                                frame 0, Default {
                                n236 = node-c288() -> (w948:T1)  [unwired: 1 in]
                                n237 = timed-loop {
                                timing: w948 -> [_]
                                timing-out: [_] -> w947
                                tunnel: w949 -> [w951]
                                stop <- TRUE stop-if-true
                                n238 = xnode ("Memory Method Node")("Address"=u32 2, "Data"=w951) -> ()  [unwired: 1 in, 1 out]
                                }
                                n239 = node-c288(w947) -> ()
                                }
                                frame 1 {
                                n240 = node-c288() -> (w958:T1)  [unwired: 1 in]
                                n241 = timed-loop {
                                timing: w958 -> [_]
                                timing-out: [_] -> w957
                                tunnel: w959 -> [w961]
                                stop <- TRUE stop-if-true
                                n242 = xnode ("Memory Method Node")("Address"=u32 2, "Data"=w961) -> ()  [unwired: 1 in, 1 out]
                                }
                                n243 = node-c288(w957) -> ()
                                }
                                frame 2 {
                                n244 = node-c288() -> (w969:T1)  [unwired: 1 in]
                                n245 = timed-loop {
                                timing: w969 -> [_]
                                timing-out: [_] -> w968
                                tunnel: w967 -> [w970]
                                stop <- TRUE stop-if-true
                                n246 = xnode ("Memory Method Node")("Address"=u32 0, "Data"=w970) -> ()  [unwired: 1 in, 1 out]
                                }
                                n247 = node-c288(w968) -> ()
                                }
                                }
                                }
                                frame #3 {
                                n248 = case shown="2" w977 {
                                tunnel: w978 -> [w981 w991 w999]
                                frame 0, Default {
                                n249 = node-c288() -> (w980:T1)  [unwired: 1 in]
                                n250 = timed-loop {
                                timing: w980 -> [_]
                                timing-out: [_] -> w979
                                tunnel: w981 -> [w983]
                                stop <- TRUE stop-if-true
                                n251 = xnode ("Memory Method Node")("Address"=u32 3, "Data"=w983) -> ()  [unwired: 1 in, 1 out]
                                }
                                n252 = node-c288(w979) -> ()
                                }
                                frame 1 {
                                n253 = node-c288() -> (w990:T1)  [unwired: 1 in]
                                n254 = timed-loop {
                                timing: w990 -> [_]
                                timing-out: [_] -> w989
                                tunnel: w991 -> [w993]
                                stop <- TRUE stop-if-true
                                n255 = xnode ("Memory Method Node")("Address"=u32 3, "Data"=w993) -> ()  [unwired: 1 in, 1 out]
                                }
                                n256 = node-c288(w989) -> ()
                                }
                                frame 2 {
                                n257 = node-c288() -> (w1001:T1)  [unwired: 1 in]
                                n258 = timed-loop {
                                timing: w1001 -> [_]
                                timing-out: [_] -> w1000
                                tunnel: w999 -> [w1002]
                                stop <- TRUE stop-if-true
                                n259 = xnode ("Memory Method Node")("Address"=u32 0, "Data"=w1002) -> ()  [unwired: 1 in, 1 out]
                                }
                                n260 = node-c288(w1000) -> ()
                                }
                                }
                                }
                                frame #4 {
                                n261 = case shown="2" w1010 {
                                tunnel: w1009 -> [w1013 w1023 w1031]
                                frame 0, Default {
                                n262 = node-c288() -> (w1012:T1)  [unwired: 1 in]
                                n263 = timed-loop {
                                timing: w1012 -> [_]
                                timing-out: [_] -> w1011
                                tunnel: w1013 -> [w1015]
                                stop <- TRUE stop-if-true
                                n264 = xnode ("Memory Method Node")("Address"=u32 4, "Data"=w1015) -> ()  [unwired: 1 in, 1 out]
                                }
                                n265 = node-c288(w1011) -> ()
                                }
                                frame 1 {
                                n266 = node-c288() -> (w1022:T1)  [unwired: 1 in]
                                n267 = timed-loop {
                                timing: w1022 -> [_]
                                timing-out: [_] -> w1021
                                tunnel: w1023 -> [w1025]
                                stop <- TRUE stop-if-true
                                n268 = xnode ("Memory Method Node")("Address"=u32 4, "Data"=w1025) -> ()  [unwired: 1 in, 1 out]
                                }
                                n269 = node-c288(w1021) -> ()
                                }
                                frame 2 {
                                n270 = node-c288() -> (w1033:T1)  [unwired: 1 in]
                                n271 = timed-loop {
                                timing: w1033 -> [_]
                                timing-out: [_] -> w1032
                                tunnel: w1031 -> [w1034]
                                stop <- TRUE stop-if-true
                                n272 = xnode ("Memory Method Node")("Address"=u32 0, "Data"=w1034) -> ()  [unwired: 1 in, 1 out]
                                }
                                n273 = node-c288(w1032) -> ()
                                }
                                }
                                }
                                frame #5 {
                                n274 = case shown="2" w1042 {
                                tunnel: w1041 -> [w1045 w1055 w1063]
                                frame 0, Default {
                                n275 = node-c288() -> (w1044:T1)  [unwired: 1 in]
                                n276 = timed-loop {
                                timing: w1044 -> [_]
                                timing-out: [_] -> w1043
                                tunnel: w1045 -> [w1047]
                                stop <- TRUE stop-if-true
                                n277 = xnode ("Memory Method Node")("Address"=u32 5, "Data"=w1047) -> ()  [unwired: 1 in, 1 out]
                                }
                                n278 = node-c288(w1043) -> ()
                                }
                                frame 1 {
                                n279 = node-c288() -> (w1054:T1)  [unwired: 1 in]
                                n280 = timed-loop {
                                timing: w1054 -> [_]
                                timing-out: [_] -> w1053
                                tunnel: w1055 -> [w1057]
                                stop <- TRUE stop-if-true
                                n281 = xnode ("Memory Method Node")("Address"=u32 5, "Data"=w1057) -> ()  [unwired: 1 in, 1 out]
                                }
                                n282 = node-c288(w1053) -> ()
                                }
                                frame 2 {
                                n283 = node-c288() -> (w1065:T1)  [unwired: 1 in]
                                n284 = timed-loop {
                                timing: w1065 -> [_]
                                timing-out: [_] -> w1064
                                tunnel: w1063 -> [w1066]
                                stop <- TRUE stop-if-true
                                n285 = xnode ("Memory Method Node")("Address"=u32 0, "Data"=w1066) -> ()  [unwired: 1 in, 1 out]
                                }
                                n286 = node-c288(w1064) -> ()
                                }
                                }
                                }
                                frame #6 {
                                n287 = xnode ("FIFO Method Node")("Element"=w1077, "Timeout"=0) -> ()  [unwired: 1 in, 2 out]
                                n288 = Increment(x=w1077) -> (x+1=w1076:u8)
                                n289 = Greater Or Equal?(x=w1076, y=u8 3) -> (x >= y?=w1078:bool)
                                n290 = Select(t=w1077, s=w1078, f=u8 0) -> (s? t:f=w1075:u8)
                                }
                                }
                              }
                            }
                            n291 = Or(x=w769, y=w768) -> (x .or. y?=w767:bool)
                          }
                          frame #3 {
                            n292 = xnode ("Register Read")() -> ("Data"=w1091:bool)  [unwired: 1 in, 1 out]
                            n293 = Less Or Equal To 0?(x=w1092) -> (x <= 0?=w1090:bool)
                            n294 = Or(x=w1091, y=w1090) -> (x .or. y?=w1089:bool)
                            n295 = case shown="False" w1089 {
                              tunnel: w1092 -> [w1100 w1114]
                              tunnel: [w1102 w1114] -> w1095
                              tunnel: fxp<+/-,48,16> 0.0048828125 ("y") -> [w1101 _]
                              tunnel: w1093 -> [w1098 _]
                              frame False {
                                n296 = xnode "High Throughput Subtract"("x"=w1100, "y"=w1098) -> ("x-y"=w1099:fxp<+/-,48,16>)
                                n297 = while {
                                shift-right: [w1107] -> w1102
                                shift-left: w1100 -> [w1113]
                                tunnel: w1101 -> [w1106]
                                tunnel: w1099 -> [w1105]
                                stop <- w1108 stop-if-true
                                n298 = xnode "High Throughput Subtract"("x"=w1113, "y"=w1106) -> ("x-y"=w1109:fxp<+/-,48,16>)
                                n299 = xnode ("Register Read")() -> ("Data"=w1112:bool)  [unwired: 1 in, 1 out]
                                n300 = Less Or Equal To 0?(x=w1109) -> (x <= 0?=w1110:bool)
                                n301 = Less Or Equal?(x=w1109, y=w1105) -> (x <= y?=w1111:bool)
                                n302 = Select(t=fxp<+/-,48,16> 0.0, s=w1110, f=w1109) -> (s? t:f=w1107:fxp<+/-,48,16>)
                                n303 = local read "RetRate us"() -> (w1103:i32)
                                n304 = xnode "FPGA I/O Node"("Connector0/AO2"=w1107) -> ()  [unwired: 1 in, 1 out]
                                n305 = Compound Arithmetic op=OR(w1110, w1111, w1112) -> (w1108:bool)
                                n306 = call "Wait11"("Count(uSec)"=w1103) -> ()  [unwired: 1 out]
                                }
                              }
                              frame True {
                              }
                            }
                          }
                        }
                      }
                      frame True {
                        n307 = xnode ("Register Read")() -> ("Data"=w1115:bool)  [unwired: 1 in, 1 out]
                        n308 = Not(x=w1118) -> (.not. x?=w1117:bool)
                        n309 = Or(x=w1117, y=w1115) -> (x .or. y?=w1116:bool)
                      }
                    }
                  }
                }
              }
            }
            frame True {
            }
          }
        }
        frame #4 {
          n310 = while {
            shift-right: [w1129] -> _
            shift-left: w1125 -> [w1134]
            tunnel: fxp<+/-,48,16> 0.0048828125 ("y") -> [w1128]
            stop <- w1130 stop-if-true
            w1126 = fxp<+/-,48,16> 0.0 ("t")
            n311 = xnode "High Throughput Subtract"("x"=w1134, "y"=w1128) -> ("x-y"=w1131:fxp<+/-,48,16>)
            n312 = Less Or Equal To 0?(x=w1131) -> (x <= 0?=w1132:bool)
            n313 = Less Or Equal?(x=w1131, y=w1126) -> (x <= y?=w1133:bool)
            n314 = Select(t=w1126, s=w1132, f=w1131) -> (s? t:f=w1129:fxp<+/-,48,16>)
            n315 = local read "RetRate us"() -> (w1127:i32)
            n316 = xnode "FPGA I/O Node"("Connector0/AO2"=w1129) -> ()  [unwired: 1 in, 1 out]
            n317 = Compound Arithmetic op=OR(w1132, w1133) -> (w1130:bool)
            n318 = call "Wait12"("Count(uSec)"=w1127) -> ()  [unwired: 1 out]
          }
          n319 = xnode "FPGA I/O Node"() -> ("Connector0/AI0"=w1123:fxp<+/-,27,5>, "Connector0/AI1"=w1122:fxp<+/-,27,5>)  [unwired: 2 in, 2 out]
        }
        frame #5 {
          n320 = call "Wait15"("Count(uSec)"=u8 100) -> ()  [unwired: 1 out]
        }
        frame #6 {
          n321 = while {
            shift-right: [w1145] -> _
            shift-left: w1138 -> [w1150]
            tunnel: fxp<+/-,48,16> 0.0048828125 ("y") -> [w1144]
            stop <- w1146 stop-if-true
            w1143 = fxp<+/-,48,16> 0.0 ("t")
            n322 = xnode "High Throughput Subtract"("x"=w1150, "y"=w1144) -> ("x-y"=w1147:fxp<+/-,48,16>)
            n323 = Less Or Equal To 0?(x=w1147) -> (x <= 0?=w1148:bool)
            n324 = Less Or Equal?(x=w1147, y=w1143) -> (x <= y?=w1149:bool)
            n325 = Select(t=w1143, s=w1148, f=w1147) -> (s? t:f=w1145:fxp<+/-,48,16>)
            n326 = xnode "FPGA I/O Node"("Connector0/AO1"=w1145) -> ()  [unwired: 1 in, 1 out]
            n327 = Compound Arithmetic op=OR(w1148, w1149) -> (w1146:bool)
            n328 = call "Wait14"("Count(uSec)"=u16 100) -> ()  [unwired: 1 out]
          }
          n329 = while {
            shift-right: [w1154] -> _
            shift-left: w1141 -> [w1159]
            tunnel: fxp<+/-,48,16> 0.0048828125 ("y") -> [w1153]
            stop <- w1155 stop-if-true
            w1152 = fxp<+/-,48,16> 0.0 ("t")
            n330 = xnode "High Throughput Subtract"("x"=w1159, "y"=w1153) -> ("x-y"=w1156:fxp<+/-,48,16>)
            n331 = Less Or Equal To 0?(x=w1156) -> (x <= 0?=w1157:bool)
            n332 = Less Or Equal?(x=w1156, y=w1152) -> (x <= y?=w1158:bool)
            n333 = Select(t=w1152, s=w1157, f=w1156) -> (s? t:f=w1154:fxp<+/-,48,16>)
            n334 = xnode "FPGA I/O Node"("Connector0/AO0"=w1154) -> ()  [unwired: 1 in, 1 out]
            n335 = Compound Arithmetic op=OR(w1157, w1158) -> (w1155:bool)
            n336 = call "Wait13"("Count(uSec)"=u16 100) -> ()  [unwired: 1 out]
          }
        }
        frame #7 {
          n337 = call "Wait16"("Count(uSec)"=u8 100) -> ()  [unwired: 1 out]
        }
        frame #8 {
          n338 = local write "ScanFinished?"(TRUE ("ScanFinished?")) -> ()
        }
      }
      n339 = while {
        stop <- w34 stop-if-true
        n340 = xnode ("Register Read")() -> ("Data"=w35:bool)  [unwired: 1 in, 1 out]
        n341 = xnode ("FIFO Method Node")() -> ("Number of Elements to Read"=w33:u32)  [unwired: 1 in, 1 out]
        n342 = local read "ScanFinished?"() -> (w36:bool)
        n343 = call "Wait8"("Count(uSec)"=u8 200 ("Count(mSec)")) -> ()  [unwired: 1 out]
        n344 = Or(x=w36, y=w35) -> (x .or. y?=w34:bool)
        n345 = Greater Than 0?(x=w33) -> (x > 0?=w32:bool)
        n346 = case shown="True" w32 {
          frame False {
          }
          frame True {
            # "push data in swapbuffer from target to host and clear buffer synchronously"
            n347 = flat-sequence {
              frame #0 {
              }
              frame #1 {
                n348 = xnode ("FIFO Method Node")("Timeout"=8192) -> ("Element"=w38:u8)  [unwired: 1 in, 2 out]
                n349 = case shown="0, Default" w38 {
                  frame 0, Default {
                    n350 = flat-sequence {
                      frame #0 {
                        n351 = node-c288(refnum<k21> "10MHz" ("Source Name")) -> (w42:T1)
                        n352 = timed-loop {
                          timing: w42 -> [_]
                          timing-out: [_] -> w41
                          shift-right: [w44] -> _
                          shift-left: _ -> [w51]
                          shift-right: [w51] -> _
                          shift-left: _ -> [w50]
                          shift-right: [w50] -> _
                          shift-left: _ -> [w47]
                          i -> [w43]
                          stop <- w48 stop-if-true
                          n353 = Greater Or Equal?(x=w43, y=16386) -> (x >= y?=w48:bool)
                          n354 = Greater Or Equal?(x=w43, y=3) -> (x >= y?=w46:bool)
                          n355 = case shown="True" w46 {
                            tunnel: w47 -> [_ w52]
                            frame False {
                            }
                            frame True {
                              n356 = xnode ("FIFO Method Node")("Element"=w52, "Timeout"=0) -> ()  [unwired: 1 in, 2 out]
                            }
                          }
                          n357 = xnode ("Memory Method Node")("Address"=w43) -> ("Data"=w44:fxp<+/-,48,16>)  [unwired: 1 in, 1 out]
                        }
                        n358 = node-c288(w41) -> ()
                      }
                      frame #1 {
                        n359 = node-c288() -> (w61:T1)  [unwired: 1 in]
                        n360 = timed-loop {
                          timing: w61 -> [_]
                          timing-out: [_] -> w60
                          i -> [w62]
                          stop <- w63 stop-if-true
                          n361 = xnode ("Memory Method Node")("Address"=w62, "Data"=fxp<+/-,48,16> -100.0) -> ()  [unwired: 1 in, 1 out]
                          n362 = Greater Or Equal?(x=w62, y=16383) -> (x >= y?=w63:bool)
                        }
                        n363 = node-c288(w60) -> ()
                      }
                    }
                  }
                  frame 1 {
                    n364 = flat-sequence {
                      frame #0 {
                        n365 = node-c288(refnum<k21> "10MHz" ("Source Name")) -> (w72:T1)
                        n366 = timed-loop {
                          timing: w72 -> [_]
                          timing-out: [_] -> w71
                          shift-right: [w81] -> _
                          shift-left: _ -> [w80]
                          shift-right: [w80] -> _
                          shift-left: _ -> [w79]
                          shift-right: [w79] -> _
                          shift-left: _ -> [w76]
                          i -> [w75]
                          stop <- w77 stop-if-true
                          n367 = Greater Or Equal?(x=w75, y=3) -> (x >= y?=w74:bool)
                          n368 = Greater Or Equal?(x=w75, y=16386) -> (x >= y?=w77:bool)
                          n369 = case shown="True" w74 {
                            tunnel: w76 -> [_ w82]
                            frame False {
                            }
                            frame True {
                              n370 = xnode ("FIFO Method Node")("Element"=w82, "Timeout"=0) -> ()  [unwired: 1 in, 2 out]
                            }
                          }
                          n371 = xnode ("Memory Method Node")("Address"=w75) -> ("Data"=w81:fxp<+/-,48,16>)  [unwired: 1 in, 1 out]
                        }
                        n372 = node-c288(w71) -> ()
                      }
                      frame #1 {
                        n373 = node-c288() -> (w91:T1)  [unwired: 1 in]
                        n374 = timed-loop {
                          timing: w91 -> [_]
                          timing-out: [_] -> w90
                          i -> [w92]
                          stop <- w94 stop-if-true
                          n375 = xnode ("Memory Method Node")("Address"=w92, "Data"=fxp<+/-,48,16> -100.0) -> ()  [unwired: 1 in, 1 out]
                          n376 = Greater Or Equal?(x=w92, y=16383) -> (x >= y?=w94:bool)
                        }
                        n377 = node-c288(w90) -> ()
                      }
                    }
                  }
                  frame 2 {
                    n378 = flat-sequence {
                      frame #0 {
                        n379 = node-c288(refnum<k21> "10MHz" ("Source Name")) -> (w102:T1)
                        n380 = timed-loop {
                          timing: w102 -> [_]
                          timing-out: [_] -> w101
                          shift-right: [w103] -> _
                          shift-left: _ -> [w111]
                          shift-right: [w111] -> _
                          shift-left: _ -> [w110]
                          shift-right: [w110] -> _
                          shift-left: _ -> [w107]
                          i -> [w104]
                          stop <- w108 stop-if-true
                          n381 = Greater Or Equal?(x=w104, y=3) -> (x >= y?=w106:bool)
                          n382 = Greater Or Equal?(x=w104, y=16386) -> (x >= y?=w108:bool)
                          n383 = case shown="True" w106 {
                            tunnel: w107 -> [_ w112]
                            frame False {
                            }
                            frame True {
                              n384 = xnode ("FIFO Method Node")("Element"=w112, "Timeout"=0) -> ()  [unwired: 1 in, 2 out]
                            }
                          }
                          n385 = xnode ("Memory Method Node")("Address"=w104) -> ("Data"=w103:fxp<+/-,48,16>)  [unwired: 1 in, 1 out]
                        }
                        n386 = node-c288(w101) -> ()
                      }
                      frame #1 {
                        n387 = node-c288() -> (w121:T1)  [unwired: 1 in]
                        n388 = timed-loop {
                          timing: w121 -> [_]
                          timing-out: [_] -> w120
                          i -> [w123]
                          stop <- w124 stop-if-true
                          n389 = xnode ("Memory Method Node")("Address"=w123, "Data"=fxp<+/-,48,16> -100.0) -> ()  [unwired: 1 in, 1 out]
                          n390 = Greater Or Equal?(x=w123, y=16383) -> (x >= y?=w124:bool)
                        }
                        n391 = node-c288(w120) -> ()
                      }
                    }
                  }
                }
              }
              frame #2 {
              }
            }
          }
        }
      }
    }
    frame #3 {
      n392 = local write "TargetDone?"(TRUE ("TargetDone?")) -> ()
    }
  }
